vi "soundwave.vi"() -> ()   [LabVIEW 2023]
panel:
  out "Waveform Graph":waveform(dbl)(graph)
  in  "Delta t (s)":dbl
  in  "Durata (s)":dbl
  in  "Ampiezza":dbl(knob) scale=1.0..5.0
  in  "Frequenza":dbl(knob) scale=200.0..1000.0
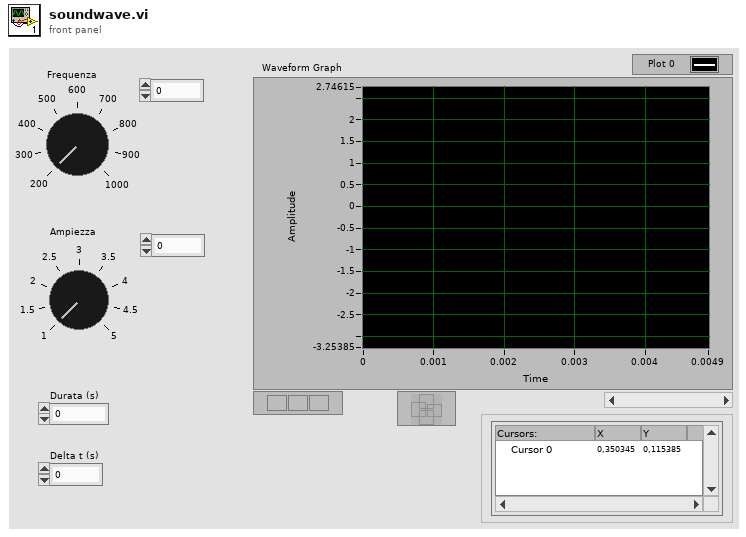
[diagram p1: front panel]
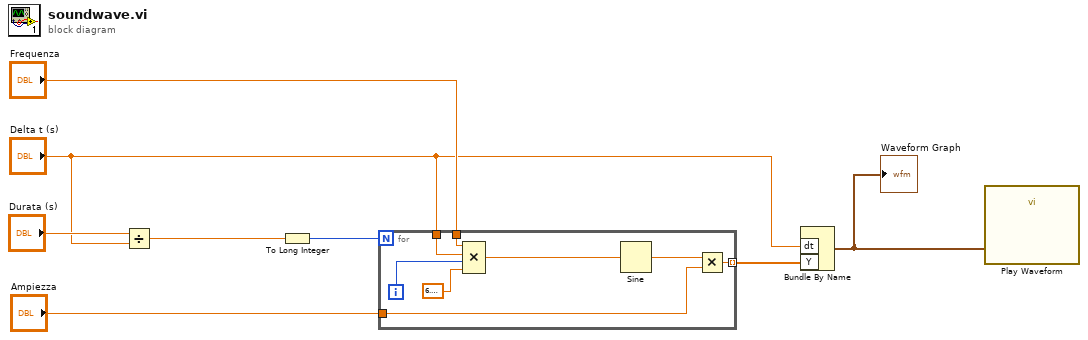
[diagram p0: block diagram]
diagram:
  n1 = Divide(x="Durata (s)", y="Delta t (s)") -> (x/y=w6:dbl)
  n2 = To Long Integer(number=w6) -> (32bit integer=w7:i32)
  n3 = for {
    N: w7 -> [_]
    tunnel: "Ampiezza" -> [w16]
    tunnel: "Frequenza" -> [w13]
    tunnel: "Delta t (s)" -> [w12]
    tunnel: [w9] -> w2 mode=indexing
    i -> [w11]
    n4 = Compound Arithmetic op=MULTIPLY(w13, w12, w11, 6.283185307179586) -> (w14:dbl)
    n5 = Sine(x=w14) -> (sin(x)=w15:dbl)
    n6 = Multiply(x=w15, y=w16) -> (x*y=w9:dbl)
  }
  n7 = Bundle By Name("dt"="Delta t (s)", "Y"=w2) -> (w1:waveform(dbl))  [unwired: 1 in]
  "Waveform Graph" <- w1
  n8 = call "Play Waveform"("Data"=w1) -> ()  [unwired: 18 in, 1 out]
